vi "7digitdisplay.vi"(5 "Numeric":dbl) -> (4 "Array":bool[](array[boolean]))   [LabVIEW 2021]
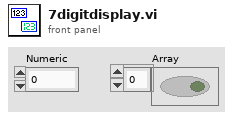
[diagram p1: front panel]
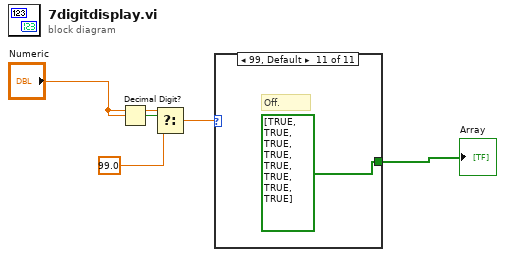
[diagram p0: block diagram]
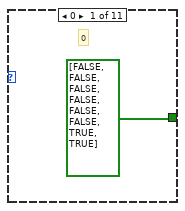
[diagram p2: hidden frame]
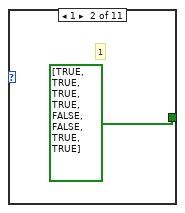
[diagram p3: hidden frame]
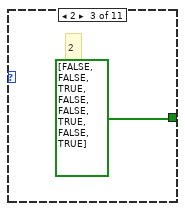
[diagram p4: hidden frame]
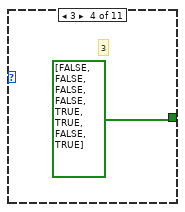
[diagram p5: hidden frame]
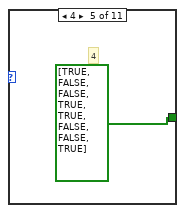
[diagram p6: hidden frame]
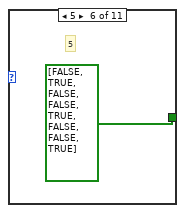
[diagram p7: hidden frame]
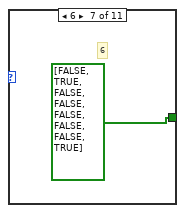
[diagram p8: hidden frame]
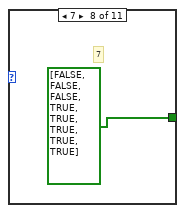
[diagram p9: hidden frame]
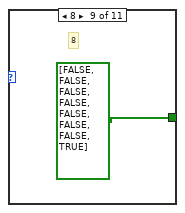
[diagram p10: hidden frame]
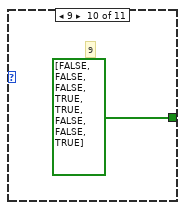
[diagram p11: hidden frame]
diagram:
  n1 = Decimal Digit?(1:"Numeric") -> (0:w4:bool)
  n2 = Select(t="Numeric", s=w4, f=99.0) -> (s? t:f=w1:dbl)
  n3 = case shown="99, Default" w1 {
    tunnel: [bool[] [FALSE, FALSE, FALSE, FALSE, FALSE, FALSE, TRUE, TRUE] bool[] [TRUE, TRUE, TRUE, TRUE, FALSE, FALSE, TRUE, TRUE] bool[] [FALSE, FALSE, TRUE, FALSE, FALSE, TRUE, FALSE, TRUE] bool[] [FALSE, FALSE, FALSE, FALSE, TRUE, TRUE, FALSE, TRUE] bool[] [TRUE, FALSE, FALSE, TRUE, TRUE, FALSE, FALSE, TRUE] bool[] [FALSE, TRUE, FALSE, FALSE, TRUE, FALSE, FALSE, TRUE] bool[] [FALSE, TRUE, FALSE, FALSE, FALSE, FALSE, FALSE, TRUE] bool[] [FALSE, FALSE, FALSE, TRUE, TRUE, TRUE, TRUE, TRUE] bool[] [FALSE, FALSE, FALSE, FALSE, FALSE, FALSE, FALSE, TRUE] bool[] [FALSE, FALSE, FALSE, TRUE, TRUE, FALSE, FALSE, TRUE] bool[] [TRUE, TRUE, TRUE, TRUE, TRUE, TRUE, TRUE, TRUE]] -> w5
    frame 0 {
      # "0"
    }
    frame 1 {
      # "1"
    }
    frame 2 {
      # "2"
    }
    frame 3 {
      # "3"
    }
    frame 4 {
      # "4"
    }
    frame 5 {
      # "5"
    }
    frame 6 {
      # "6"
    }
    frame 7 {
      # "7"
    }
    frame 8 {
      # "8"
    }
    frame 9 {
      # "9"
    }
    frame 99, Default {
      # "Off."
    }
  }
  "Array" <- w5
